vi "add alarm comparison.vi"(5 "Limit":dbl, 7 "comparison":T2, 8 "error in":errorcluster, 9 "data type":T1, 10 "alarm name":string, 11 "alarms module configuration in":refnum<class "alarms module configuration.lvclass">) -> (0 "error out":errorcluster, 1 "created channels":refnum<class "TBM channel.lvclass">[](array[class]), 2 "compare index":i32, 3 "alarms module configuration out":refnum<class "alarms module configuration.lvclass">)   [LabVIEW 2013, in "alarms module configuration.lvclass"]
uses:
  alarms module configuration.lvclass
  compare type.ctl
  <vilib>/NI/Tag Bus Module Framework/channel/TBM channel.lvclass
  <vilib>/NI/Tag Bus/tag/Data Type.ctl
  alarms module configuration.lvclass/alarms module configuration.ctl
  alarm comparison.ctl
  <vilib>/NI/Tag Bus Module Framework/channel/channel classification.ctl
  <vilib>/NI/Configuration Framework/serializable configuration/NISE_CEF_serializable configuration.lvclass
  <vilib>/NI/Tag Bus/tag/tag descriptor.lvclass
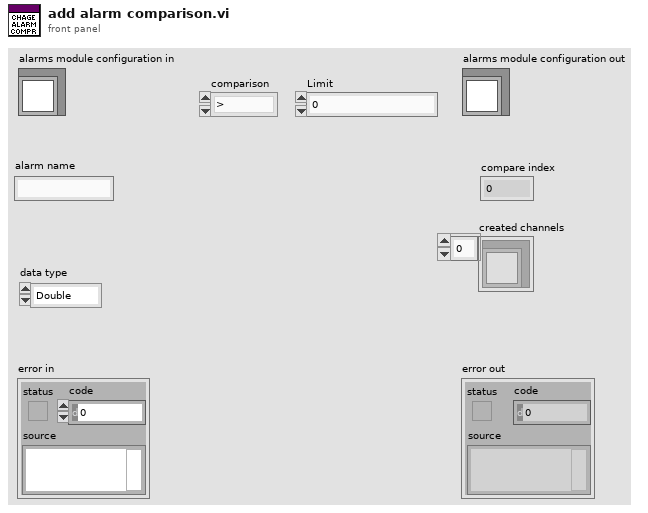
[diagram p1: front panel]
types:
  T1 = typedef "tag bus.lvlib/tag descriptor.lvclass/Data Type.ctl" = enum16{"Double", "Single", "I64", "I32", "I16", "I8", "U64", "U32", "U16", "U8", "Boolean", "String", "Array of Double", "Array of Single", "Array of I64", "Array of I32", "Array of I16", "Array of I8", "Array of U64", "Array of U32", "Array of U16", "Array of U8", "Array of Boolean", "Array of String"}
  T2 = typedef "alarms module configuration.lvclass/compare type.ctl" = enum16{">", "<", ">=", "<=", "="}
  T3 = typedef "TBM channel.lvclass/channel classification.ctl" = enum16{"input data", "output data", "processing parameter", "processing result"}
  T4 = typedef "alarms module configuration.lvclass/alarm comparison.ctl" = cluster{"input channel":refnum<class "TBM channel.lvclass">, "limit":dbl, "comparison":T2}
  T5 = typedef "alarms module configuration.lvclass/alarm configuration.ctl" = cluster{"alarm name":string, "comparisons":T4[], "unlatch":refnum<class "TBM channel.lvclass">, "output":refnum<class "TBM channel.lvclass">, "boolean op":T6}
  T6 = typedef "alarms module configuration.lvclass/boolean operation.ctl" = enum16{"AND", "OR"}
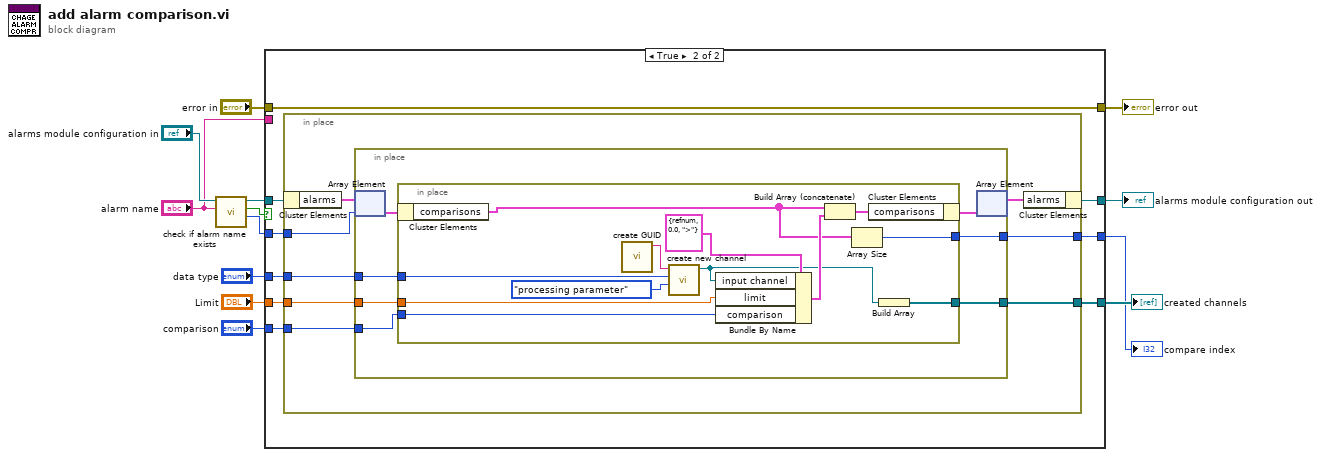
[diagram p0: block diagram]
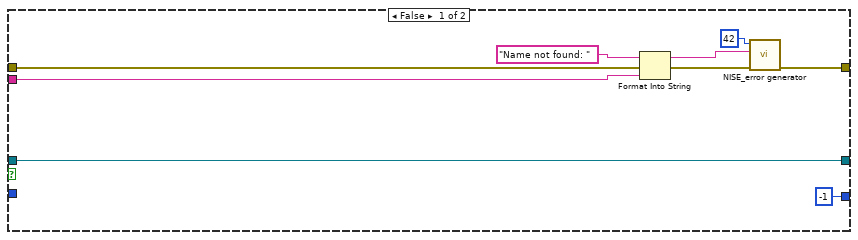
[diagram p2: hidden frame]
diagram:
  n1 = call "check if alarm name exists.vi"("name to locate"="alarm name", "alarms module configuration in"="alarms module configuration in") -> ("index"=w7:i32, "found?"=w10:bool, "alarms module configuration out"=w8:refnum<class "alarms module configuration.lvclass">)  [unwired: 6 in, 1 out]
  n2 = case shown="True" w10 {
    tunnel: [w21 w29] -> w12
    tunnel: "error in" -> [w22 w29]
    tunnel: [w16 w30] -> w9
    tunnel: w8 -> [w16 w31]
    tunnel: w7 -> [_ w28]
    tunnel: "alarm name" -> [w15 _]
    tunnel: "Limit" -> [_ w27]
    tunnel: "comparison" -> [_ w26]
    tunnel: "data type" -> [_ w25]
    tunnel: [_ w24] -> w2
    tunnel: [-1 w23] -> w1
    frame False {
      n3 = Format Into String(initial string="Name not found: " ("append error message"), error in=w22, w15) -> (resulting string=w17:string, error out=w19:errorcluster)  [unwired: 1 in]
      n4 = call <vilib>:"NISE_error generator.vi"("error in"=w19, "append error message"=w17, "error code (0)"=42) -> ("error out"=w21:errorcluster)  [unwired: 6 in]
    }
    frame True {
      n5 = in-place {
        in-place-border: w28 -> [w37]
        in-place-border: w27 -> [w36]
        in-place-border: w26 -> [w35]
        in-place-border: w25 -> [w34]
        in-place-border: [w33] -> w24
        in-place-border: [w32] -> w23
        n6 = in-place-cluster #1(w31) -> ("alarms"=w39:T5[])
        n7 = in-place {
          in-place-border: w36 -> [w45]
          in-place-border: w35 -> [w44]
          in-place-border: w34 -> [w42]
          in-place-border: [w41] -> w33
          in-place-border: [w40] -> w32
          n8 = in-place-array #2(w39, w37) -> (w46:T5)
          n9 = in-place {
            in-place-border: w45 -> [w58]
            in-place-border: w44 -> [w57]
            in-place-border: w42 -> [w51]
            in-place-border: [w49] -> w41
            in-place-border: [w47] -> w40
            n10 = in-place-cluster #3(w46) -> ("comparisons"=w48:T4[])
            n11 = call <vilib>:"create GUID.vi"() -> ("uuid"=w53:string)  [unwired: 10 in, 1 out]
            n12 = call <vilib>:"create new channel.vi"("channel classification"=channel_classification."processing parameter", "data type"=w51, "channel name"=w53) -> ("channel"=w50:refnum<class "TBM channel.lvclass">)  [unwired: 8 in]
            n13 = Bundle By Name(cluster=T4 {"input channel"=refnum, "limit"=0.0, "comparison"=enum.">"} ("element"), "input channel"=w50, "limit"=w58, "comparison"=w57) -> (w54:T4)
            n14 = Build Array (concatenate)(w48, w54) -> (w55:T4[])
            n15 = Array Size(array=w48) -> (size(s)=w47:i32)
            n16 = in-place-cluster #3("comparisons"=w55) -> (w43:T5)
            n17 = Build Array(w50) -> (w49:refnum<class "TBM channel.lvclass">[])
          }
          n18 = in-place-array #2(w43) -> (w38:T5[])  [unwired: 1 out]
        }
        n19 = in-place-cluster #1("alarms"=w38) -> (w30:refnum<class "alarms module configuration.lvclass">)
      }
    }
  }
  "error out" <- w12
  "alarms module configuration out" <- w9
  "compare index" <- w1
  "created channels" <- w2
